vi "sort.vi"(0 "Output length":i32, 1 "Real":sgl[](array[numeric])=[0.0, 0.0, 0.0, 0.0, 0.0, 0.0, 0.0, 0.0, 0.0, 0.0, 0.0, 0.0, 0.0, 0.0, 0.0, 0.0, 0.0, 0.0, 0.0, 0.0], 2 "Img":sgl[](array[numeric])=[0.0, 0.0, 0.0, 0.0, 0.0, 0.0, 0.0, 0.0, 0.0, 0.0, 0.0, 0.0, 0.0, 0.0, 0.0, 0.0, 0.0, 0.0, 0.0, 0.0], 3 "n":i32) -> (7 "Sorted Real":sgl[](array[numeric]), 8 "Sorted Img":sgl[](array[numeric]), 9 "Index":i32[](array[numeric]))   [LabVIEW 2020]
uses:
  <vilib>/rvi/Emulation/niFpgaGetClockAttributes.vi
  <vilib>/rvi/Emulation/niFpgaSctlEmulationGetInTimedLoop.vi
  <vilib>/rvi/Emulation/niFpgaEmulationReportErrorSimple.vi
  <vilib>/rvi/Emulation/niFpgaCriticalErrorInLSC.vi
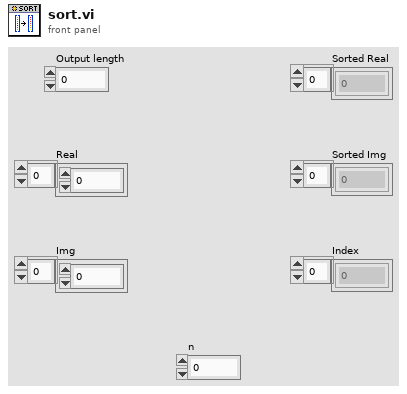
[diagram p1: front panel]
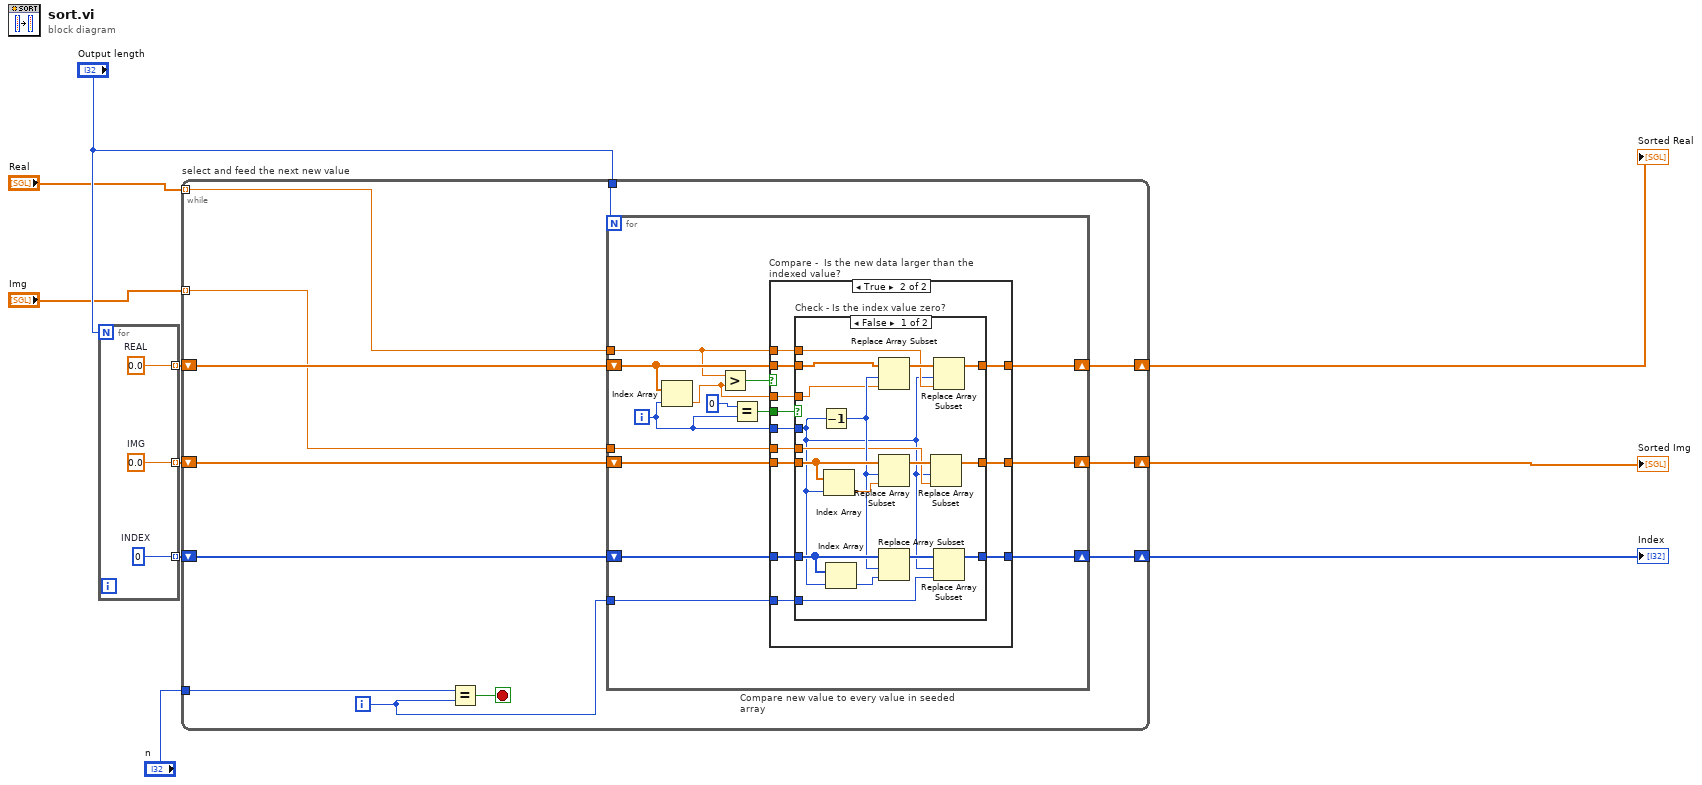
[diagram p0: block diagram]
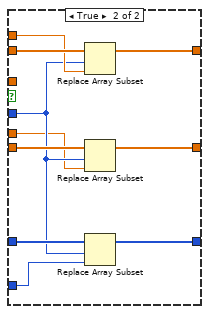
[diagram p3: hidden frame]
diagram:
  n1 = for {
    N: "Output length" -> [_]
    tunnel: [w13] -> w4 mode=indexing
    tunnel: [w12] -> w5 mode=indexing
    tunnel: [w11] -> w6 mode=indexing
    w11 = sgl 0.0  # IMG
    w12 = 0  # INDEX
    w13 = sgl 0.0  # REAL
  }
  n2 = while "select and feed the next new value" {
    shift-right: [w24] -> w7
    shift-left: w4 -> [w25]
    shift-right: [w23] -> w9
    shift-left: w5 -> [w22]
    tunnel: "Output length" -> [w21]
    tunnel: "n" -> [w19]
    shift-right: [w17] -> w8
    shift-left: w6 -> [w16]
    tunnel: "Real" -> [w15] mode=indexing
    tunnel: "Img" -> [w14] mode=indexing
    i -> [w20]
    stop <- w18 stop-if-true
    n3 = Equal?(x=w19, y=w20) -> (x = y?=w18:bool)
    n4 = for "Compare new value to every value in seeded array" {
      N: w21 -> [_]
      tunnel: w15 -> [w37]
      shift-right: [w36] -> w24
      shift-left: w25 -> [w38]
      tunnel: w20 -> [w34]
      shift-right: [w32] -> w23
      shift-left: w22 -> [w33]
      shift-right: [w29] -> w17
      shift-left: w16 -> [w28]
      tunnel: w14 -> [w27]
      i -> [w35]
      n5 = Index Array(array=w38, index=w35) -> (element=w26:sgl)
      n6 = Greater?(x=w37, y=w26) -> (0:w39:bool)
      n7 = Equal?(x=0, y=w35) -> (x = y?=w30:bool)
      n8 = case "Compare -  Is the new data larger than the indexed value?" shown="True" w39 {
        tunnel: w38 -> [w42 w53]
        tunnel: w30 -> [_ w54]
        tunnel: w37 -> [_ w52]
        tunnel: w35 -> [_ w51]
        tunnel: [w42 w50] -> w36
        tunnel: w34 -> [_ w49]
        tunnel: w33 -> [w41 w48]
        tunnel: [w41 w47] -> w32
        tunnel: [w40 w46] -> w29
        tunnel: w28 -> [w40 w45]
        tunnel: w27 -> [_ w44]
        tunnel: w26 -> [_ w43]
        frame False {
        }
        frame True {
          n9 = case "Check - Is the index value zero?" shown="False" w54 {
            tunnel: w53 -> [w57 w81]
            tunnel: w52 -> [w70 w80]
            tunnel: w51 -> [w56 w74]
            tunnel: [w69 w79] -> w50
            tunnel: w49 -> [w64 w78]
            tunnel: w48 -> [w66 w77]
            tunnel: [w65 w76] -> w47
            tunnel: [w59 w72] -> w46
            tunnel: w45 -> [w63 w75]
            tunnel: w44 -> [w58 w73]
            tunnel: w43 -> [w55 _]
            frame False {
              n10 = Decrement(x=w56) -> (x-1=w61:i32)
              n11 = Index Array(array=w63, index=w56) -> (element=w62:sgl)
              n12 = Index Array(array=w66, index=w56) -> (element=w68:i32)
              n13 = Replace Array Subset(array=w57, new element=w55, index=w61) -> (w71:sgl[])
              n14 = Replace Array Subset(array=w63, new element=w62, index=w61) -> (w60:sgl[])
              n15 = Replace Array Subset(array=w66, new element=w68, index=w61) -> (w67:i32[])
              n16 = Replace Array Subset(array=w60, new element=w58, index=w56) -> (w59:sgl[])
              n17 = Replace Array Subset(array=w71, new element=w70, index=w56) -> (w69:sgl[])
              n18 = Replace Array Subset(array=w67, new element=w64, index=w56) -> (w65:i32[])
            }
            frame True {
              n19 = Replace Array Subset(array=w81, new element=w80, index=w74) -> (w79:sgl[])
              n20 = Replace Array Subset(array=w75, new element=w73, index=w74) -> (w72:sgl[])
              n21 = Replace Array Subset(array=w77, new element=w78, index=w74) -> (w76:i32[])
            }
          }
        }
      }
    }
  }
  "Index" <- w9
  "Sorted Img" <- w8
  "Sorted Real" <- w7
